vi "Loop.vi"(10 "Actor":refnum<class "Actor.lvclass">) -> ()   [LabVIEW 2021, in "Queue Actor.lvclass"]
uses:
  Queue Actor.lvclass
  Actor/Actor.lvclass
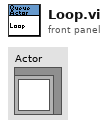
[diagram p1: front panel]
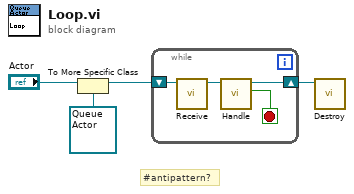
[diagram p0: block diagram]
diagram:
  # "#antipattern?"
  n1 = To More Specific Class(target class=refnum<class "Queue Actor.lvclass"> refnum ("Queue Actor.lvclass"), reference="Actor") -> (specific class reference=w2:refnum<class "Queue Actor.lvclass">)  [unwired: 1 in, 1 out]
  n2 = while {
    shift-right: [w8] -> w4
    shift-left: w2 -> [w6]
    stop <- w7 stop-if-true
    n3 = call-dynamic "Receive.vi"("Queue Actor in"=w6) -> ("Queue Actor out"=w5:refnum<class "Queue Actor.lvclass">)  [unwired: 10 in]
    n4 = call-dynamic "Handle.vi"("Queue Actor in"=w5) -> ("Destroy?"=w7:bool, "Queue Actor out"=w8:refnum<class "Queue Actor.lvclass">)  [unwired: 9 in]
  }
  n5 = call-dynamic "Destroy.vi"("Queue Actor in"=w4) -> ()  [unwired: 11 in]
